vi "WriteFloatParameter.vi"(3 "Value":sgl, 4 "Address":u32, 5 "Device":u8=1, 6 "Serial port":refnum<visa-resource-name>) -> (2 "Serial port out":refnum<visa-resource-name>)   [LabVIEW 2021]
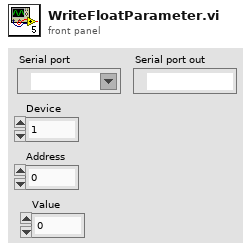
[diagram p1: front panel]
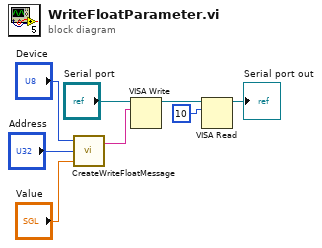
[diagram p0: block diagram]
diagram:
  n1 = call "CreateWriteFloatMessage.vi"("Value"="Value", "Address"="Address", "Device"="Device") -> ("Message"=w1:string)  [unwired: 1 in]
  n2 = VISA Write(VISA resource name="Serial port", write buffer=w1) -> (VISA resource name out=w8:refnum<visa-resource-name>)  [unwired: 1 in, 2 out]
  n3 = VISA Read(VISA resource name=w8, byte count=u32 10) -> (VISA resource name out=→"Serial port out":refnum<visa-resource-name>)  [unwired: 1 in, 3 out]
